vi "Write Root Node.vi"(8 "error in":errorcluster, 10 "Root Node":variant, 11 "config-base in":refnum<class "config-base.lvclass">) -> (0 "error out":errorcluster, 3 "config-base out":refnum<class "config-base.lvclass">)   [LabVIEW 2022 SP3, in "hse-config.lvlib" / "config-base.lvclass"]
doc: "____\nHAMPEL SOFTWARE ENGINEERING v3.8.0 (2023-12-18 14:41)"
uses:
  config-base.lvclass
  config-base.lvclass/config-base.ctl
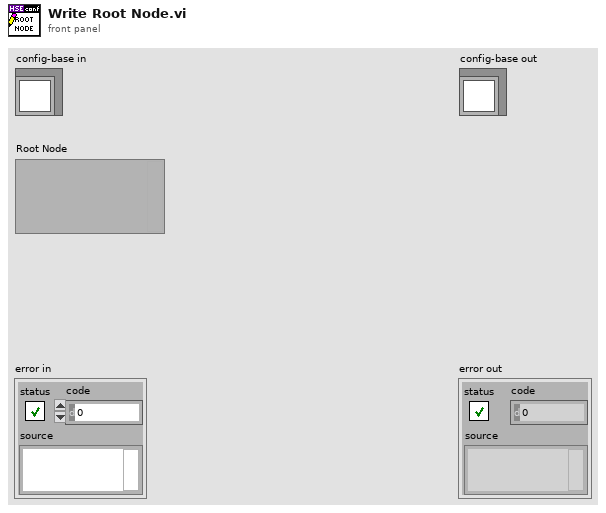
[diagram p1: front panel]
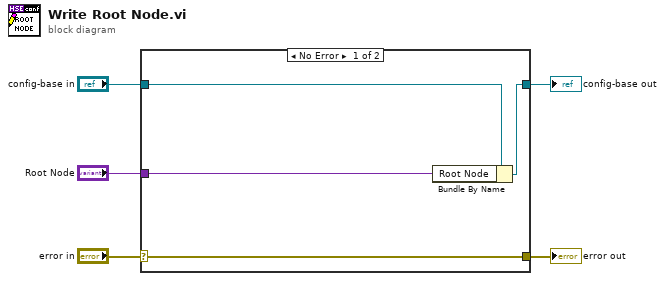
[diagram p0: block diagram]
diagram:
  n1 = case shown="No Error" "error in" {
    selector: "error in" -> [w9 w10]
    tunnel: [w9 w10] -> w4
    tunnel: [w7 w11] -> w2
    tunnel: "config-base in" -> [w8 w11]
    tunnel: "Root Node" -> [w6 _]
    frame No Error {
      n2 = Bundle By Name(cluster=w8, "Root Node"=w6) -> (w7:refnum<class "config-base.lvclass">)
    }
    frame Error {
    }
  }
  "error out" <- w4
  "config-base out" <- w2
